vi "Ando OSA.vi"() -> ()   [LabVIEW 2011]
uses:
  <vilib>/Utility/file.llb/Write To Spreadsheet File (I64).vi
  <vilib>/Utility/file.llb/Write To Spreadsheet File (DBL).vi
panel:
  in  "export path 2":path=path "E:/XuYi"
  out "Time array":dbl[](array[numeric])=[3.0, 170907.0, 194700.0]
  in  "filename root":string="EOM_comb" caption="File Name"
  in  "seconds to wait":u32=60
  in  "stop":bool
  out "XY Graph":cluster{"Wavelength":sgl[], "Level":sgl[]}(graph)
  out "Error Out":errorcluster
  in  "Error In":errorcluster
  in  "Trace (0:A)":enum16{"A", "B", "C"}(ring)
  in  "VISA session":refnum<visa-resource-name>="GPIB0::1::INSTR"
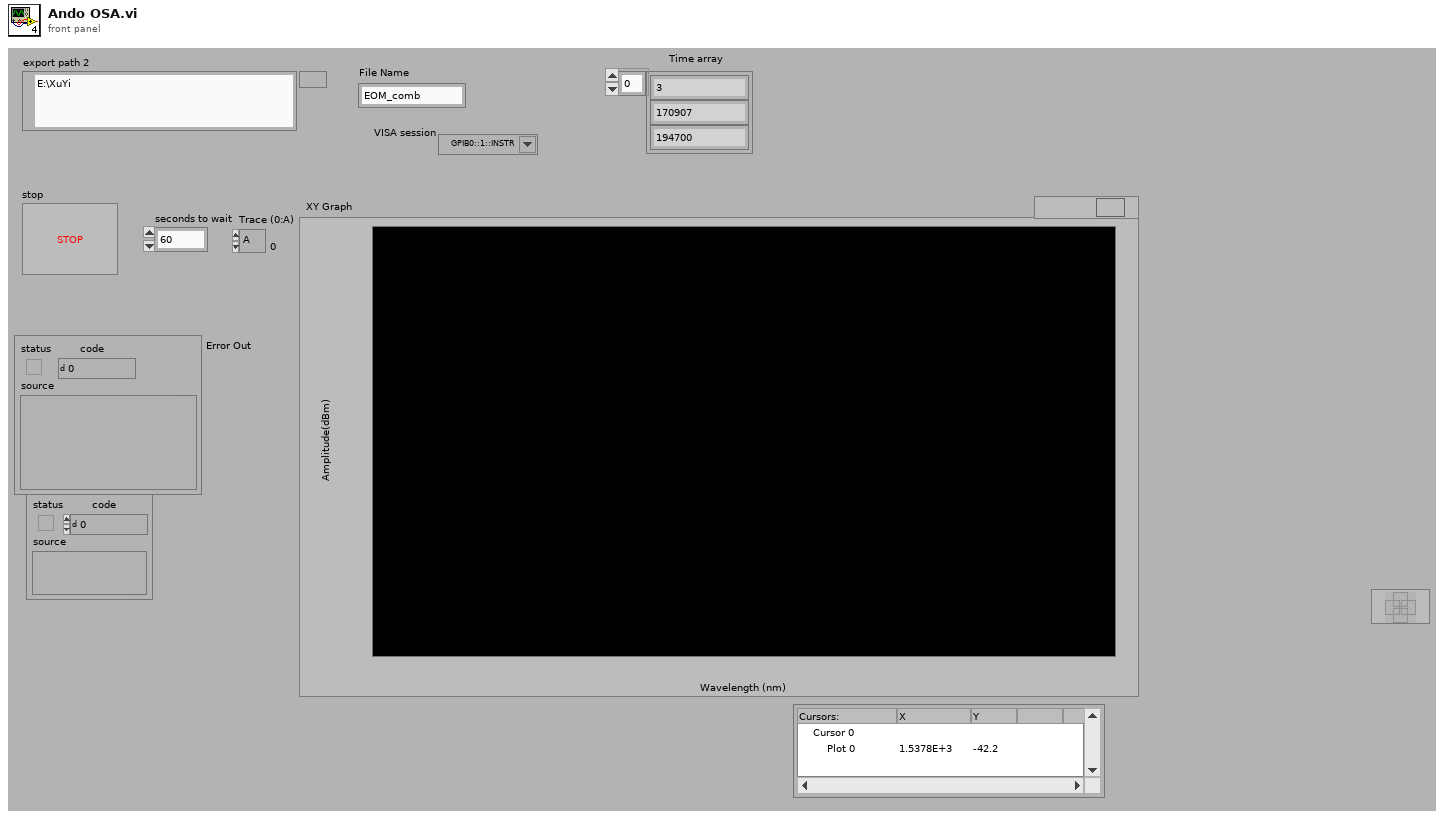
[diagram p1: front panel]
types:
  T1 = typedef "imagedata.ctl" = cluster{"image type":i32, "image depth":i32, "image":u8[], "mask":u8[], "colors":u32[], "Rectangle":cluster{"left":i16, "top":i16, "right":i16, "bottom":i16}}
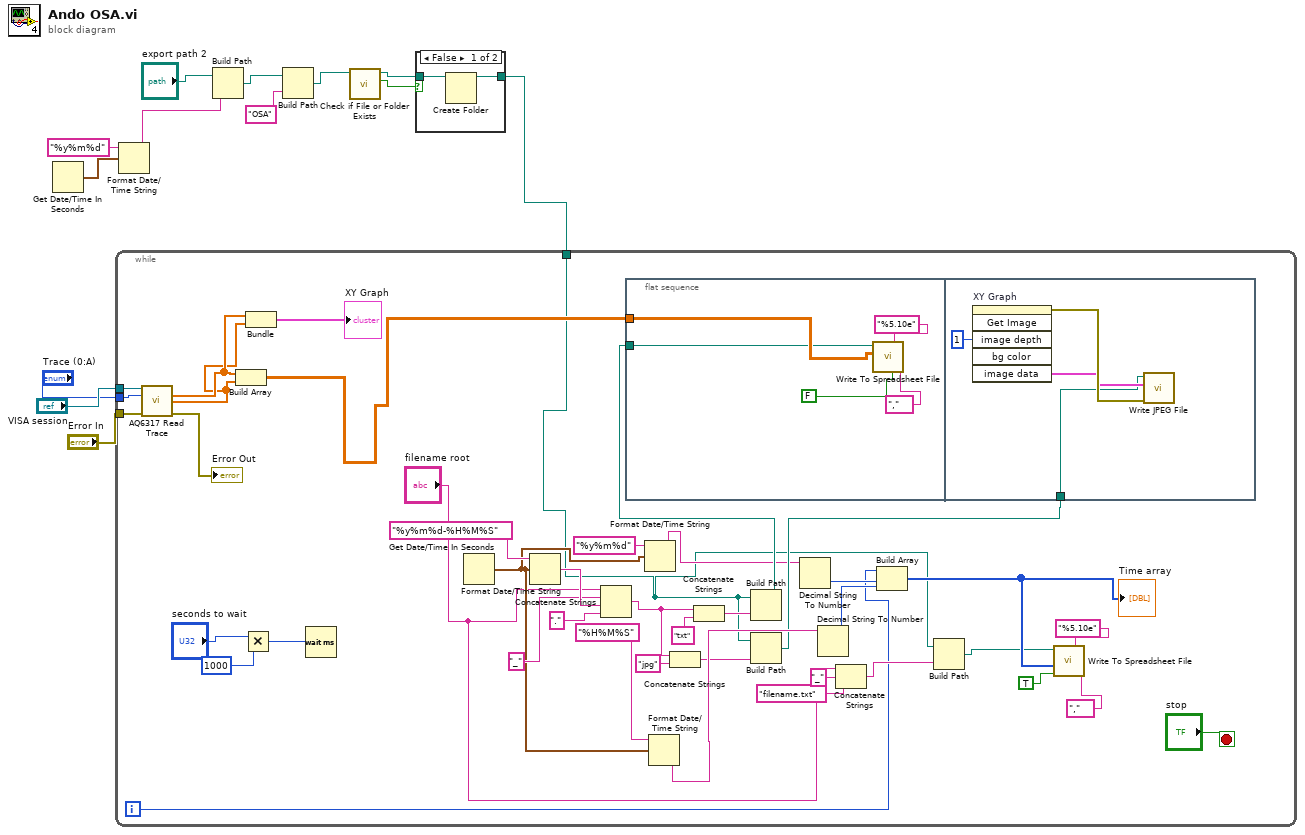
[diagram p0: block diagram]
diagram:
  n1 = Get Date/Time In Seconds() -> (seconds since 1Jan1904=w9:timestamp)
  n2 = Format Date/Time String(time format string (%c)="%y%m%d", seconds (now)=w9) -> (date/time string=w8:string)  [unwired: 1 in]
  n3 = Build Path(base path="export path 2", name or relative path=w8) -> (appended path=w4:path)
  n4 = Build Path(base path=w4, name or relative path="OSA") -> (appended path=w3:path)
  n5 = call <vilib>:"Check if File or Folder Exists.vi"("path"=w3) -> ("file or folder exists?"=w5:bool, "dup path"=w6:path)  [unwired: 8 in, 1 out]
  n6 = case shown="False" w5 {
    tunnel: [w15 w16] -> w1
    tunnel: w6 -> [w14 w16]
    frame False {
      n7 = Create Folder(path (use dialog)=w14) -> (created path=w15:path)  [unwired: 2 in, 2 out]
    }
    frame True {
    }
  }
  n8 = while {
    tunnel: "VISA session" -> [w57]
    tunnel: "Trace (0:A)" -> [w56]
    tunnel: "Error In" -> [w55]
    tunnel: w1 -> [w17]
    i -> [w28]
    stop <- "stop" stop-if-true
    n9 = call <instrlib>:"AQ6317 Read Trace.vi"("VISA session"=w57, "Trace (0:A)"=w56, "Error In"=w55) -> ("Wavelength"=w52:sgl[], "Level"=w51:sgl[], "Error Out"=→"Error Out":errorcluster)  [unwired: 7 in, 3 out]
    n10 = Build Array(w52, w51) -> (w53:sgl[][])
    n11 = Multiply(x="seconds to wait", y=u32 1000) -> (x*y=w46:u32)
    n12 = Bundle("Wavelength"=w52, "Level"=w51) -> (→"XY Graph":cluster{"Wavelength":sgl[], "Level":sgl[]})  [unwired: 1 in]
    n13 = Wait (ms)(milliseconds to wait=w46) -> ()  [unwired: 1 out]
    n14 = Get Date/Time In Seconds() -> (seconds since 1Jan1904=w36:timestamp)
    n15 = Format Date/Time String(time format string (%c)="%y%m%d-%H%M%S" ("time format string"), seconds (now)=w36) -> (date/time string=w44:string)  [unwired: 1 in]
    n16 = Concatenate Strings("filename root", "_" ("separator (_)"), w44, "." ("string")) -> (w22:string)
    n17 = flat-sequence {
      tunnel: w53 -> [w62]
      tunnel: w23 -> [w58]
      tunnel: w19 -> [w64]
      frame #0 {
        n18 = call-poly <vilib>:"Write To Spreadsheet File.vi"("delimiter (\\t)"="," ("delimiter (Tab)"), "transpose? (no:F)"=FALSE, "format (%.3f)"="%5.10e", "2D data"=w62, "file path (dialog if empty)"=w58) -> ()  [unwired: 3 in, 1 out]
      }
      frame #1 {
        n19 = invoke on="XY Graph" class="XYGraph (strict)" method="Get Image"("image depth"=1 ("Image Depth")) -> (error out=w66:errorcluster, "image data"=w65:T1)  [unwired: 5 in, 4 out]
        n20 = call <vilib>:"Write JPEG File.vi"("error in (no error)"=w66, "image data"=w65, "path to JPEG file"=w64) -> ()  [unwired: 7 in, 2 out]
      }
    }
    n21 = Format Date/Time String(time format string (%c)="%y%m%d", seconds (now)=w36) -> (date/time string=w18:string)  [unwired: 1 in]
    n22 = Format Date/Time String(time format string (%c)="%H%M%S", seconds (now)=w36) -> (date/time string=w27:string)  [unwired: 1 in]
    n23 = Concatenate Strings(w22, "jpg" ("string")) -> (w20:string)
    n24 = Concatenate Strings(w22, "txt" ("extension")) -> (w24:string)
    n25 = Build Path(base path=w17, name or relative path=w24) -> (appended path=w23:path)
    n26 = Build Path(base path=w17, name or relative path=w20) -> (appended path=w19:path)
    n27 = Decimal String To Number(string=w18) -> (number=w29:i32)  [unwired: 2 in, 1 out]
    n28 = Decimal String To Number(string=w27) -> (number=w30:i32)  [unwired: 2 in, 1 out]
    n29 = Concatenate Strings("filename root", "_" ("string"), "filename.txt" ("string")) -> (w31:string)
    n30 = Build Array(w28, w29, w30) -> (w40:i32[])
    "Time array" <- w40
    n31 = Build Path(base path=w17, name or relative path=w31) -> (appended path=w35:path)
    n32 = call-poly <vilib>:"Write To Spreadsheet File.vi"("delimiter (\\t)"="," ("delimiter (Tab)"), "format (%d)"="%5.10e" ("format (%.3f)"), "append to file? (new file:F)"=TRUE ("transpose? (no:F)"), "1D data"=w40, "file path (dialog if empty)"=w35) -> ()  [unwired: 3 in, 1 out]
  }
